vi "setKey.vi"(4 "Alignment":cluster{"Horizontal":string, "Vertical":string}, 6 "Appearance":T2, 8 "Set?":bool=TRUE, 9 "\"At\" location":T1, 10 "Location":string(combo)="auto", 11 "String in":string) -> (1 "command":string, 3 "String out":string)   [LabVIEW 2012]
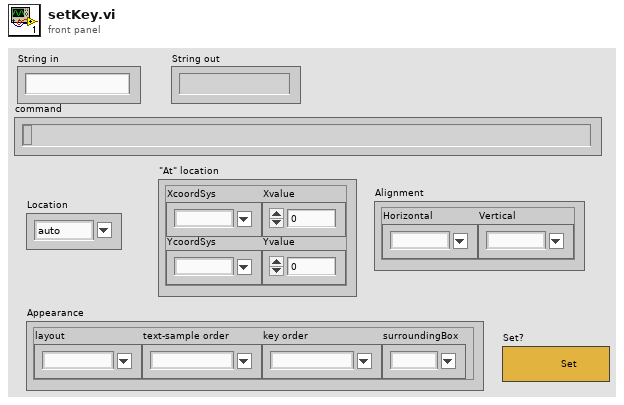
[diagram p1: front panel]
types:
  T1 = cluster{"XcoordSys":string, "YcoordSys":string, "Xvalue":dbl, "Yvalue":dbl}
  T2 = cluster{"layout":string, "text-sample order":string, "key order":string, "surroundingBox":string}
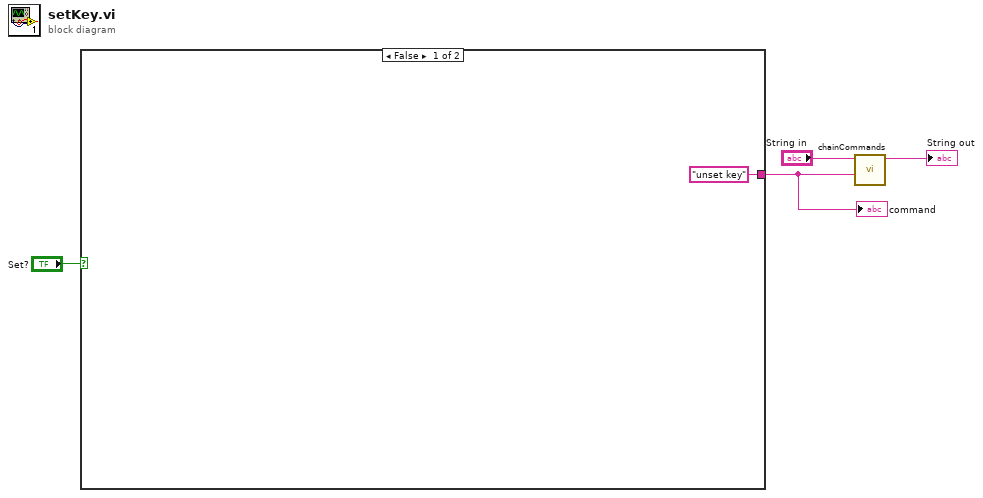
[diagram p0: block diagram]
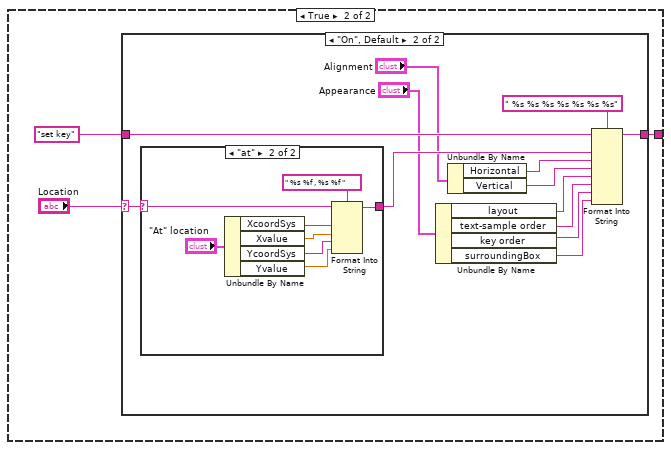
[diagram p2: hidden frame]
diagram:
  n1 = case shown="False" "Set?" {
    tunnel: ["unset key" w6] -> w2
    frame False {
    }
    frame True {
      n2 = case shown="\"On\", Default" "Location" {
        selector: "Location" -> [_ w19]
        tunnel: [w9 w22] -> w6
        tunnel: "set key" -> [w9 w21]
        frame "auto" {
        }
        frame "On", Default {
          n3 = case shown="\"at\"" w19 {
            selector: w19 -> [w23 w31]
            tunnel: [w23 w30] -> w18
            frame "False", Default {
            }
            frame "at" {
              n4 = Unbundle By Name("\"At\" location") -> ("XcoordSys"=w28:string, "Xvalue"=w27:dbl, "YcoordSys"=w26:string, "Yvalue"=w25:dbl)
              n5 = Format Into String(format string=" %s %f , %s %f ", initial string=w31, w28, w27, w26, w25) -> (resulting string=w30:string)  [unwired: 1 in, 1 out]
            }
          }
          n6 = Unbundle By Name("Appearance") -> ("layout"=w12:string, "text-sample order"=w16:string, "key order"=w15:string, "surroundingBox"=w14:string)
          n7 = Unbundle By Name("Alignment") -> ("Horizontal"=w10:string, "Vertical"=w11:string)
          n8 = Format Into String(format string=" %s %s %s %s %s %s %s", initial string=w21, w18, w10, w11, w12, w16, w15, w14) -> (resulting string=w22:string)  [unwired: 1 in, 1 out]
        }
      }
    }
  }
  "command" <- w2
  n9 = call "chainCommands.vi"("Command"=w2, "StringIn"="String in") -> ("StringOut"=→"String out":string)  [unwired: 9 in]
